vi "InitJoy.vi"(8 "error in (no error)":errorcluster, 10 "device index":i32, 11 "Joystick in":refnum<class "Joystick.lvclass">) -> (0 "error out":errorcluster, 3 "Joystick out":refnum<class "Joystick.lvclass">)   [LabVIEW 2014, in "Joystick.lvclass"]
uses:
  Joystick.lvclass
  Joystick.lvclass/Joystick.ctl
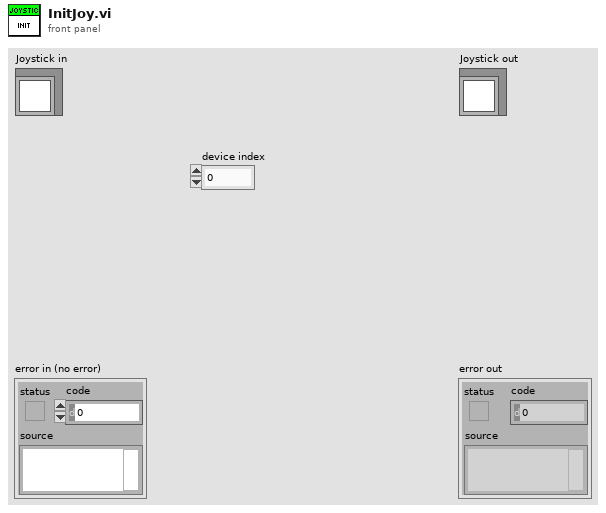
[diagram p1: front panel]
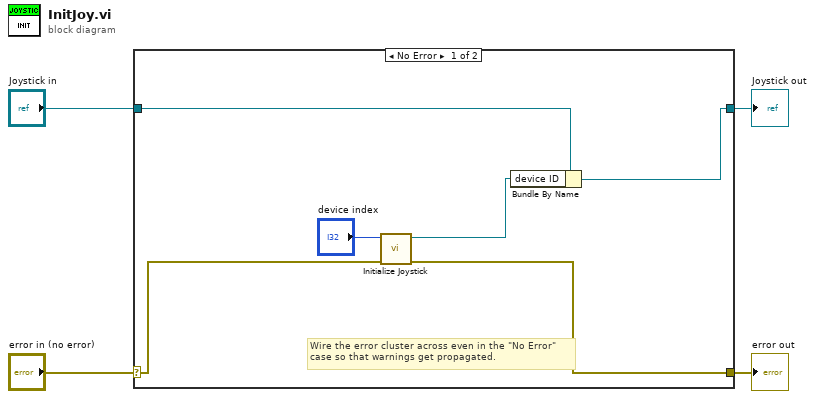
[diagram p0: block diagram]
diagram:
  n1 = case shown="No Error" "error in (no error)" {
    selector: "error in (no error)" -> [w6 w12]
    tunnel: [w5 w12] -> w3
    tunnel: [w8 w11] -> w1
    tunnel: "Joystick in" -> [w9 w11]
    frame No Error {
      # "Wire the error cluster across even in the \"No Error\"\ncase so that warnings get propagated."
      n2 = call <vilib>:"Initialize Joystick.vi"("error in (no error)"=w6, "device index"="device index") -> ("error out"=w5:errorcluster, "device ID"=w7:refnum<k1>)  [unwired: 8 in]
      n3 = Bundle By Name(cluster=w9, "device ID"=w7) -> (w8:refnum<class "Joystick.lvclass">)
    }
    frame Error {
    }
  }
  "error out" <- w3
  "Joystick out" <- w1
